vi "ws_edittest export sequence.vi"(6 "User":T1, 8 "error in (no error)":errorcluster, 10 "Sequence ID":string, 11 "Connection Refnum":T2) -> (0 "error out":errorcluster, 2 "Exported Sequence":string, 3 "Connection Refnum":T2)   [LabVIEW 2011]
uses:
  SI.LIB/ODBC/SQL Controls/Connection Refnum.ctl
  server/database/Users/User Record.ctl
  <vilib>/Utility/config.llb/NI_LVConfig.lvlib
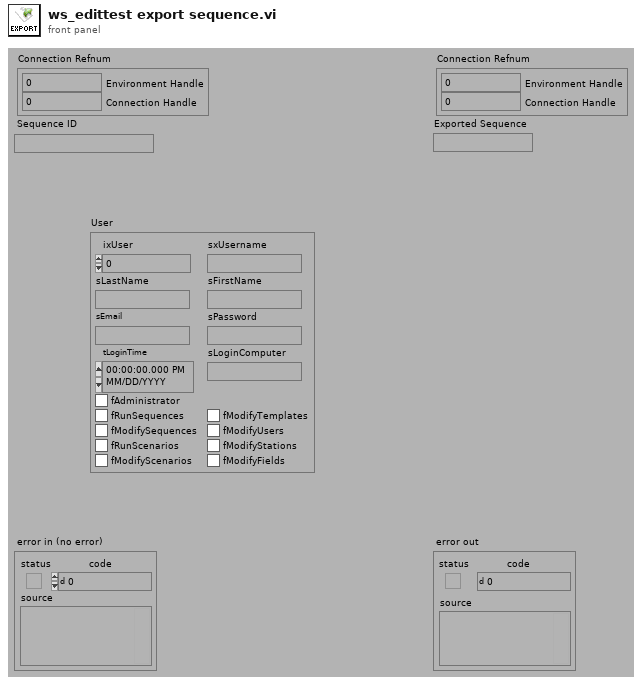
[diagram p1: front panel]
types:
  T1 = typedef "User Record.ctl" = cluster{"ixUser":i32, "sxUsername":string, "sLastName":string, "sFirstName":string, "sEmail":string, "sPassword":string, "tLoginTime":timestamp, "sLoginComputer":string, "fAdministrator":bool, "fRunSequences":bool, "fModifySequences":bool, "fRunScenarios":bool, "fModifyScenarios":bool, "fModifyTemplates":bool, "fModifyUsers":bool, "fModifyStations":bool, "fModifyFields":bool}
  T2 = typedef "Connection Refnum.ctl" = cluster{"Environment Handle":i32, "Connection Handle":i32}
  T3 = typedef "Sequence Record.ctl" = cluster{"ixSequence":i32, "sxSequenceId":string, "sDescription":string, "sCreator":string, "tCreationDate":timestamp, "sModifier":string, "tModifiedDate":timestamp, "fApproved":bool, "fSpartanSetsSN":bool, "fOverwriteData":bool, "fStopOnFail":bool, "fDisableQuickMode":bool, "fPartialExecution":bool, "fAutoNextItem":bool, "fDoNotPrintOnFail":bool}
  T4 = typedef "Step Record.ctl" = cluster{"ixStep":i32, "sxSequenceId":string, "sxTestId":string, "iIndex":i32, "iRepeat":i32, "iQuickMode":i32, "sTag":string, "sDatasheetsCSV":string, "bConfiguration":string}
  T5 = typedef "Field Record.ctl" = cluster{"ixField":i32, "iSequenceOrder":i32, "sxFieldId":string, "sxSequenceId":string, "sDisplayName":string, "sValue":string, "sUnits":string, "nDataType":T6, "nNextItem":T7, "fSystem":bool, "fSystemValue":bool, "fRequired":bool, "fSetAtTest":bool, "fTestField":bool, "fDeleted":bool, "fIndexed":bool, "fFreeList":bool}
  T6 = typedef "Field DataTypes.ctl" = enum32{"text", "numeric", "list", "timestamp", "boolean"}
  T7 = typedef "Field NextItem.ctl" = enum32{"Reset", "Retain", "Auto-Increment"}
  T8 = typedef "OGAB Version.ctl" = cluster{"Version":string, "Build Number":u32, "Build Date/Time":dbl}
  T9 = typedef "NI_LVConfig.lvlib/Config Data RefNum.ctl" = refnum<k1>
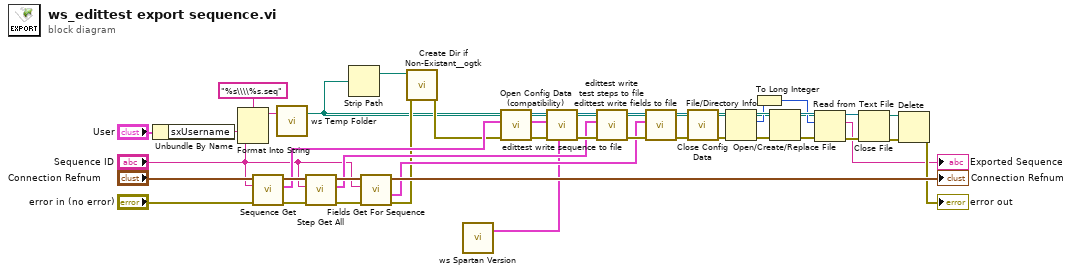
[diagram p0: block diagram]
diagram:
  n1 = Unbundle By Name("User") -> ("sxUsername"=w20:string)
  n2 = Format Into String(format string="%s\\\\%s.seq" ("Relative Path (\"\" - Folder)"), w20, "Sequence ID") -> (resulting string=w22:string)  [unwired: 2 in, 1 out]
  n3 = call "Sequence Get.vi"("error in (no error)"="error in (no error)", "sxSequenceId (\"\")"="Sequence ID", "Connection Refnum"="Connection Refnum") -> ("error out"=w39:errorcluster, "Sequence Record"=w31:T3, "Connection Refnum"=w36:T2)  [unwired: 6 out]
  n4 = call "ws Temp Folder.vi"("Relative Path (\"\")"=w22) -> ("Temp Folder"=w2:path)  [unwired: 2 in]
  n5 = call "Step Get All.vi"("error in (no error)"=w39, "sxSequenceId"="Sequence ID", "Connection Refnum"=w36) -> ("error out"=w37:errorcluster, "Sequence Steps"=w28:T4[], "Connection Refnum"=w35:T2)  [unwired: 1 in, 5 out]
  n6 = Strip Path(path=w2) -> (stripped path=w16:path)  [unwired: 1 out]
  n7 = call "Fields Get For Sequence.vi"("error in (no error)"=w37, "sxSequenceId (\"\")"="Sequence ID", "Connection Refnum"=w35) -> ("error out"=w17:errorcluster, "Current Sequence Fields"=w18:T5[], "Connection Refnum"=→"Connection Refnum":T2)  [unwired: 6 out]
  n8 = call <userlib>:"Create Dir if Non-Existant__ogtk.vi"("error in (no error)"=w17, "Directory Path"=w16) -> ("error out"=w15:errorcluster)  [unwired: 1 in, 8 out]
  n9 = call "ws Spartan Version.vi"() -> ("Version"=w1:T8)  [unwired: 3 in]
  n10 = call <vilib>:"Open Config Data (compatibility).vi"("error in (no error)"=w15, "configuration file path"=w2) -> ("error out"=w33:errorcluster, "refnum"=w32:T9)  [unwired: 7 in, 1 out]
  n11 = call "edittest write sequence to file.vi"("Spartan Version"=w1, "error in (no error)"=w33, "Sequence Record"=w31, "File Refnum In"=w32) -> ("error out"=w30:errorcluster, "File Refnum Out"=w29:T9)  [unwired: 6 out]
  n12 = call "edittest write test steps to file.vi"("error in (no error)"=w30, "Sequence Steps"=w28, "File Refnum In"=w29) -> ("error out"=w27:errorcluster, "File Refnum Out"=w26:T9)  [unwired: 7 out]
  n13 = call "edittest write fields to file.vi"("error in (no error)"=w27, "Sequence Fields"=w18, "File Refnum In"=w26) -> ("error out"=w24:errorcluster, "File Refnum Out"=w25:T9)  [unwired: 7 out]
  n14 = call <vilib>:"Close Config Data.vi"("error in (no error)"=w24, "refnum"=w25) -> ("error out"=w14:errorcluster)  [unwired: 1 in, 8 out]
  n15 = File/Directory Info(path=w2, error in=w14) -> (path out=w12:path, size=w11:i64, error out=w13:errorcluster)  [unwired: 4 out]
  n16 = To Long Integer(number=w11) -> (32bit integer=w8:i32)
  n17 = Open/Create/Replace File(file path (use dialog)=w12, error in=w13) -> (refnum out=w10:refnum<file>, error out=w9:errorcluster)  [unwired: 5 out]
  n18 = Read from Text File(file (use dialog)=w10, count=w8, error in=w9) -> (refnum out=w6:refnum<file>, text=→"Exported Sequence":string, error out=w7:errorcluster)  [unwired: 2 out]
  n19 = Close File(refnum=w6, error in=w7) -> (error out=w5:errorcluster)  [unwired: 1 out]
  n20 = Delete(path (use dialog)=w2, error in=w5) -> (error out=→"error out":errorcluster)  [unwired: 5 out]
